vi "Mercury_GoToField_SubVI.vi"(8 "error in (no error)":errorcluster, 11 "Mercury Targets":T1) -> (0 "error out":errorcluster)   [LabVIEW 2013]
doc: "USE AT YOUR OWN RISK!\nThis subVI is meant to be called as a subVI of \"Mercury_GoToField.vi\", which will take care of the persistent switch for you"
panel:
  # "USE AT YOUR OWN RISK!\nThis subVI is meant to be called as a subVI of \"Mercury_GoToField.vi\", which will take care of the persistent switch for you"
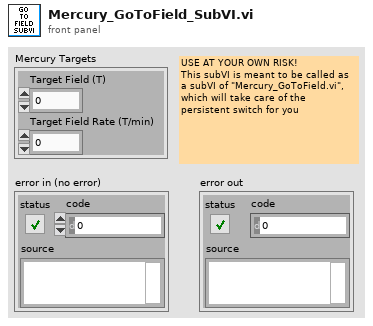
[diagram p1: front panel]
types:
  T1 = cluster{"Target Field (T)":dbl, "Target Field Rate (T/min)":dbl}
  T2 = cluster{"Hold":bool, "Clamp":bool, "To Set":bool, "To Zero":bool, "Send to IPS":bool, "PS Heat":bool, "Lambda":bool}
  T3 = cluster{"Magnet Field":dbl, "PS Field":dbl, "Target Field":dbl, "Target Field Rate":dbl, "Voltage":dbl, "Current":dbl, "Switch":bool}
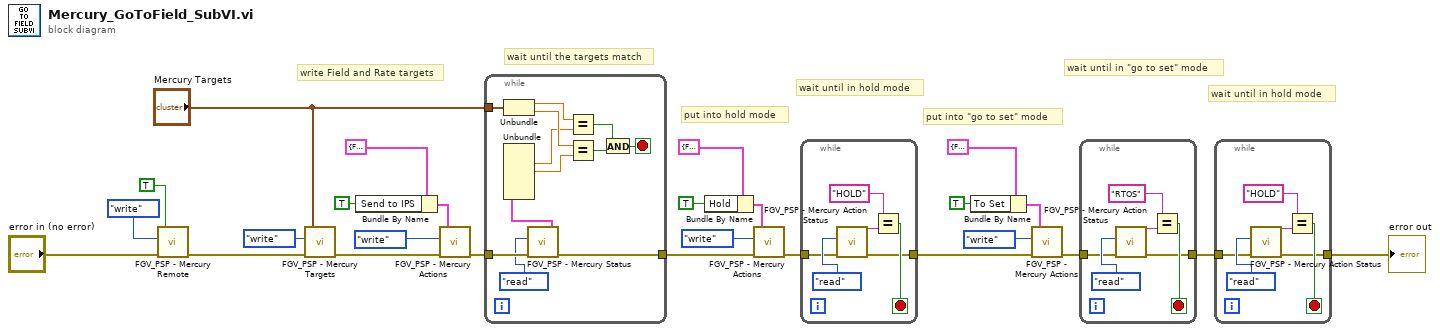
[diagram p0: block diagram]
diagram:
  # "wait until in hold mode"
  # "wait until in \"go to set\" mode"
  # "put into \"go to set\" mode"
  # "wait until in hold mode"
  # "put into hold mode"
  # "wait until the targets match"
  # "write Field and Rate targets"
  n1 = call "FGV_PSP - Mercury Remote.vi"("error in"="error in (no error)", "Function"=enum16{"write", "read"}."write", "Mercury Remote"=TRUE) -> ("error out"=w2:errorcluster)  [unwired: 3 in, 1 out]
  n2 = call "FGV_PSP - Mercury Targets.vi"("error in"=w2, "Function"=enum16{"write", "read"}."write", "Mercury Targets"="Mercury Targets") -> ("error out"=w19:errorcluster)  [unwired: 3 in, 1 out]
  n3 = Bundle By Name(cluster=T2 {"Hold"=FALSE, "Clamp"=FALSE, "To Set"=FALSE, "To Zero"=FALSE, "Send to IPS"=FALSE, "PS Heat"=FALSE, "Lambda"=FALSE} ("mercury actions"), "Send to IPS"=TRUE) -> (w18:T2)
  n4 = call "FGV_PSP - Mercury Actions.vi"("error in"=w19, "Function"=enum16{"write", "read"}."write", "mercury actions"=w18) -> ("error out"=w20:errorcluster)  [unwired: 3 in, 1 out]
  n5 = while {
    tunnel: w20 -> [w38]
    tunnel: "Mercury Targets" -> [w37]
    tunnel: [w33] -> w23
    stop <- w36 stop-if-true
    n6 = Unbundle(w37) -> ("Target Field (T)"=w35:dbl, "Target Field Rate (T/min)"=w34:dbl)
    n7 = call "FGV_PSP - Mercury Status.vi"("error in"=w38, "Function"=enum16{"write", "read"}."read") -> ("error out"=w33:errorcluster, "status"=w27:T3)  [unwired: 4 in]
    n8 = Unbundle(w27) -> ("Target Field"=w28:dbl, "Target Field Rate"=w29:dbl)  [unwired: 5 out]
    n9 = Equal?(x=w35, y=w28) -> (x = y?=w30:bool)
    n10 = Equal?(x=w34, y=w29) -> (x = y?=w31:bool)
    n11 = And(x=w30, y=w31) -> (x .and. y?=w36:bool)
  }
  n12 = Bundle By Name(cluster=T2 {"Hold"=FALSE, "Clamp"=FALSE, "To Set"=FALSE, "To Zero"=FALSE, "Send to IPS"=FALSE, "PS Heat"=FALSE, "Lambda"=FALSE} ("mercury actions"), "Hold"=TRUE ("Send to IPS")) -> (w10:T2)
  n13 = call "FGV_PSP - Mercury Actions.vi"("error in"=w23, "Function"=enum16{"write", "read"}."write", "mercury actions"=w10) -> ("error out"=w22:errorcluster)  [unwired: 3 in, 1 out]
  n14 = while {
    tunnel: w22 -> [w40]
    tunnel: [w39] -> w24
    stop <- w42 stop-if-true
    n15 = call "FGV_PSP - Mercury Action Status.vi"("error in"=w40, "Function"=enum16{"write", "read"}."read") -> ("error out"=w39:errorcluster, "Mercury Status 2"=w44:string)  [unwired: 4 in]
    n16 = Equal?(x="HOLD", y=w44) -> (x = y?=w42:bool)
  }
  n17 = Bundle By Name(cluster=T2 {"Hold"=FALSE, "Clamp"=FALSE, "To Set"=FALSE, "To Zero"=FALSE, "Send to IPS"=FALSE, "PS Heat"=FALSE, "Lambda"=FALSE} ("mercury actions"), "To Set"=TRUE ("Send to IPS")) -> (w9:T2)
  n18 = call "FGV_PSP - Mercury Actions.vi"("error in"=w24, "Function"=enum16{"write", "read"}."write", "mercury actions"=w9) -> ("error out"=w14:errorcluster)  [unwired: 3 in, 1 out]
  n19 = while {
    tunnel: w14 -> [w46]
    tunnel: [w45] -> w26
    stop <- w48 stop-if-true
    n20 = call "FGV_PSP - Mercury Action Status.vi"("error in"=w46, "Function"=enum16{"write", "read"}."read") -> ("error out"=w45:errorcluster, "Mercury Status 2"=w50:string)  [unwired: 4 in]
    n21 = Equal?(x="RTOS", y=w50) -> (x = y?=w48:bool)
  }
  n22 = while {
    tunnel: w26 -> [w52]
    tunnel: [w51] -> w25
    stop <- w54 stop-if-true
    n23 = call "FGV_PSP - Mercury Action Status.vi"("error in"=w52, "Function"=enum16{"write", "read"}."read") -> ("error out"=w51:errorcluster, "Mercury Status 2"=w56:string)  [unwired: 4 in]
    n24 = Equal?(x="HOLD", y=w56) -> (x = y?=w54:bool)
  }
  "error out" <- w25
